vi "Converte Hexadecimal - Floating Point IEEE 754.vi"(1 "Par de registradores":u16[](array[numeric])) -> (0 "Floating point":sgl)   [LabVIEW 2019]
doc: "Transforma 2 words [u16] de 16 bits em um float single precision segundo a norma IEEE 754"
panel:
  out "output array":bool[](array[boolean])
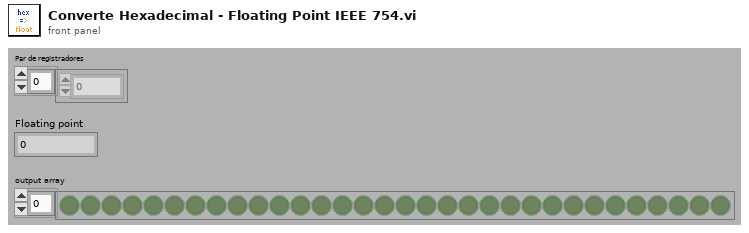
[diagram p1: front panel]
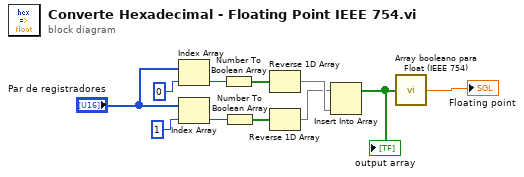
[diagram p0: block diagram]
diagram:
  n1 = Index Array(array="Par de registradores", index=0) -> (element=w2:u16)
  n2 = Index Array(array="Par de registradores", index=1) -> (element=w3:u16)
  n3 = Number To Boolean Array(number=w2) -> (Boolean array=w9:bool[])
  n4 = Number To Boolean Array(number=w3) -> (Boolean array=w8:bool[])
  n5 = Reverse 1D Array(array=w9) -> (reversed array=w6:bool[])
  n6 = Reverse 1D Array(array=w8) -> (reversed array=w5:bool[])
  n7 = Insert Into Array(array=w5, new element=w6) -> (w7:bool[])  [unwired: 1 in]
  "output array" <- w7
  n8 = call "Array booleano para Float (IEEE 754).vi"("Array [32]"=w7) -> ("Float [SGL]"=→"Floating point":sgl)
